vi "Set XY Graph To Check Delta T.vi"(9 "Cameras Number":i32, 11 "XY Graph Reference In":refnum<vi>) -> (3 "XY Graph Reference Out":refnum<vi>)   [LabVIEW 2024]
uses:
  Set XY Graph Bar Color.vi
  Set XY Graph Bar Style.vi
  Set XY Graph Interpolation Style.vi
  Set XY Graph Point Style.vi
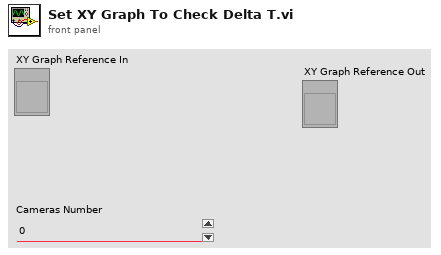
[diagram p1: front panel]
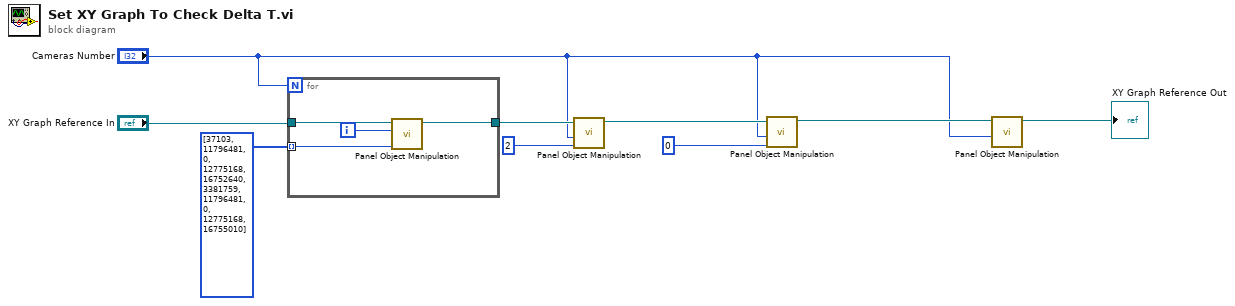
[diagram p0: block diagram]
diagram:
  n1 = for {
    N: "Cameras Number" -> [_]
    tunnel: "XY Graph Reference In" -> [w13]
    tunnel: [w12] -> w8
    tunnel: u32[] [37103, 11796481, 0, 12775168, 16752640, 3381759, 11796481, 0, 12775168, 16755010] -> [w10] mode=indexing
    i -> [w11]
    n2 = call-poly "Panel Object Manipulation.vi"("Color"=w10, "Active Plot Start"=w11, "XY Graph Reference In"=w13) -> ("XY Graph Reference Out"=w12:refnum<vi>)  [unwired: 8 in]
  }
  n3 = call-poly "Panel Object Manipulation.vi"("Bar Style"=u8 2, "Number"="Cameras Number", "XY Graph Reference In"=w8) -> ("XY Graph Reference Out"=w6:refnum<vi>)  [unwired: 8 in]
  n4 = call-poly "Panel Object Manipulation.vi"("InterPolation Style"=u8 0 ("Bar Style"), "Number"="Cameras Number", "XY Graph Reference In"=w6) -> ("XY Graph Reference Out"=w4:refnum<vi>)  [unwired: 8 in]
  n5 = call-poly "Panel Object Manipulation.vi"("Number"="Cameras Number", "XY Graph Reference In"=w4) -> ("XY Graph Reference Out"=→"XY Graph Reference Out":refnum<vi>)  [unwired: 9 in]
